vi "Show Error.vi"(4 "Error In":errorcluster, 5 "Stop Button":string="Stop", 6 "Continue/Ok Button":string="Continue", 7 "Action":T1(ring)) -> (0 "error out":errorcluster, 3 "What's Next":enum16{"Continue", "Stop"}(ring))   [LabVIEW 2015, in "Error Reporting and Storage.lvlib"]
uses:
  Error Reporting and Storage.lvlib
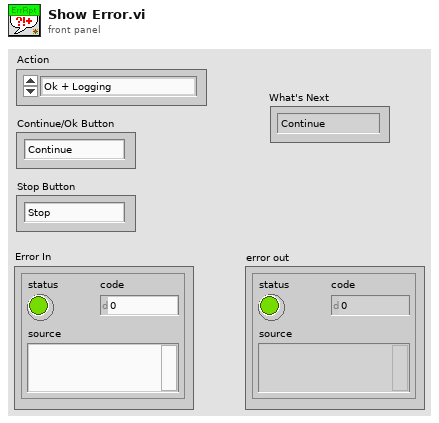
[diagram p1: front panel]
types:
  T1 = enum16{"Ok + Logging", "Continue/Stop + Logging", "Logging Only", "Ok Only", "Continue/Stop Only"}
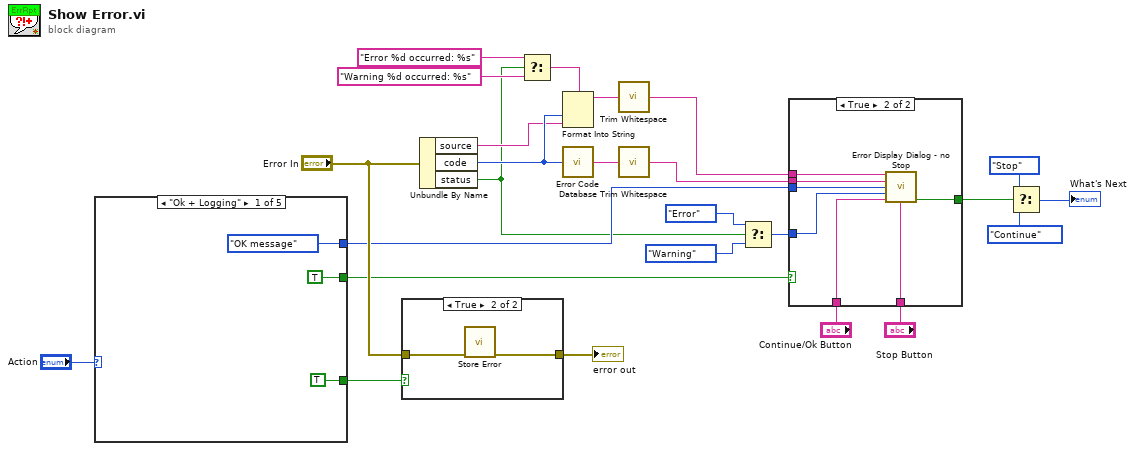
[diagram p0: block diagram]
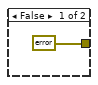
[diagram p2: hidden frame]
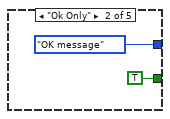
[diagram p3: hidden frame]
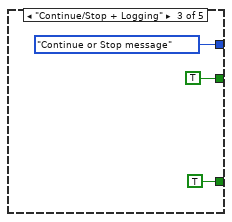
[diagram p4: hidden frame]
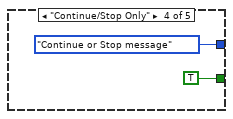
[diagram p5: hidden frame]
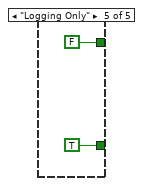
[diagram p6: hidden frame]
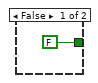
[diagram p7: hidden frame]
diagram:
  n1 = case shown="\"Ok + Logging\"" "Action" {
    tunnel: [enum16{"OK message", "Continue or Stop message"}."OK message" ("dialog type") enum16{"OK message", "Continue or Stop message"}."OK message" ("dialog type") enum16{"OK message", "Continue or Stop message"}."Continue or Stop message" ("dialog type") enum16{"OK message", "Continue or Stop message"}."Continue or Stop message" ("dialog type") _] -> w6
    tunnel: [TRUE _ TRUE _ TRUE] -> w14
    tunnel: [TRUE TRUE TRUE TRUE FALSE] -> w5
    frame "Ok + Logging" {
    }
    frame "Ok Only" {
    }
    frame "Continue/Stop + Logging" {
    }
    frame "Continue/Stop Only" {
    }
    frame "Logging Only" {
    }
  }
  n2 = case shown="True" w14 {
    tunnel: "Error In" -> [_ w40]
    tunnel: [errorcluster {"status"=FALSE, "code"=0, "source"=""} ("error out") w39] -> w12
    frame False {
    }
    frame True {
      n3 = call "Store Error.vi"("error in (no error)"=w40) -> ("error out"=w39:errorcluster)  [unwired: 6 in]
    }
  }
  "error out" <- w12
  n4 = Unbundle By Name("Error In") -> ("source"=w18:string, "code"=w20:i32, "status"=w4:bool)
  n5 = Select(t="Error %d occurred: %s" ("Error %d occurred at %s"), s=w4, f="Warning %d occurred: %s" ("Warning %d occurred at %s")) -> (s? t:f=w22:string)
  n6 = Format Into String(format string=w22, w20, w18) -> (resulting string=w24:string)  [unwired: 2 in, 1 out]
  n7 = call <vilib>:"Error Code Database.vi"("Error Code"=w20) -> ("Error Text"=w21:string)
  n8 = call <vilib>:"Trim Whitespace.vi"("string"=w24) -> ("trimmed string"=w7:string)  [unwired: 1 in]
  n9 = call <vilib>:"Trim Whitespace.vi"("string"=w21) -> ("trimmed string"=w8:string)  [unwired: 1 in]
  n10 = Select(t=enum16{"Error", "Warning"}."Error" ("Icon to Show"), s=w4, f=enum16{"Error", "Warning"}."Warning" ("Icon to Show")) -> (s? t:f=w3:enum16{"Error", "Warning"})
  n11 = case shown="True" w5 {
    tunnel: [FALSE ("stop event propagated") w42] -> w17
    tunnel: "Continue/Ok Button" -> [_ w44]
    tunnel: "Stop Button" -> [_ w43]
    tunnel: w7 -> [_ w48]
    tunnel: w8 -> [_ w47]
    tunnel: w6 -> [_ w46]
    tunnel: w3 -> [_ w45]
    frame False {
    }
    frame True {
      n12 = call "Error Display Dialog - no Stop.vi"("Source"=w48, "Details"=w47, "dialog type"=w46, "Icon to Show"=w45, "contname"=w44, "stopname"=w43) -> ("stop event propagated"=w42:bool)  [unwired: 9 in]
    }
  }
  n13 = Select(t=enum16{"Continue", "Stop"}."Stop" ("What's Next"), s=w17, f=enum16{"Continue", "Stop"}."Continue" ("What's Next")) -> (s? t:f=→"What's Next":enum16{"Continue", "Stop"})
